vi "Generate-Command-SubVI.vi"(8 "Wheel Speed":u8, 10 "Wheel Selection":u8 max=1, 11 "Wheel Position":u8) -> (3 "type":string)   [LabVIEW 2014]
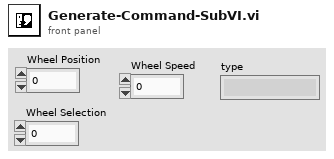
[diagram p1: front panel]
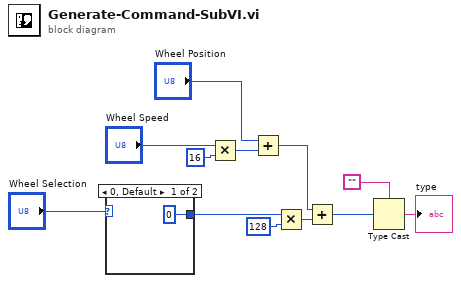
[diagram p0: block diagram]
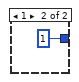
[diagram p2: hidden frame]
diagram:
  n1 = case shown="0, Default" "Wheel Selection" {
    tunnel: [0 1] -> w1
    frame 0, Default {
    }
    frame 1 {
    }
  }
  n2 = Multiply(x="Wheel Speed", y=16) -> (x*y=w9:i32)
  n3 = Add(x="Wheel Position", y=w9) -> (x+y=w4:u8)
  n4 = Multiply(x=w1, y=128) -> (x*y=w5:i32)
  n5 = Add(x=w4, y=w5) -> (x+y=w3:u8)
  n6 = Type Cast(type="", x=w3) -> (*(type *) &x=→"type":string)
